vi "Test Set Balance.vi"(8 "error in (no error)":errorcluster, 11 "Test Case In":refnum<class "Account Database Test.lvclass">) -> (0 "error out":errorcluster, 3 "Test Case Out":refnum<class "Account Database Test.lvclass">)   [LabVIEW 2020, in "Account Database Test.lvclass"]
uses:
  Account Database Test.lvclass
  C:/Program Files (x86)/National Instruments/LabVIEW 2020/vi.lib/Astemes/LUnit/Test Case.lvclass
  <vilib>/Astemes/LUnit/Test Case.lvclass/Test Case.ctl
  323c7dbb-e18d-4710-9182-97262e8b68d0.vi
  <vilib>/Astemes/LUnit/Palette/Pass.vi
  <vilib>/Astemes/LUnit/Palette/Fail.vi
  <vilib>/Astemes/LUnit/Compare Variants.vi
  <vilib>/Astemes/LUnit/Describe Comparison.vi
  <vilib>/Astemes/LUnit/Set Assertion Type.vi
  <vilib>/Astemes/LUnit/Add test result.vi
  <vilib>/Astemes/LUnit/Variant to string.vi
  <vilib>/Astemes/LUnit/LUnit Record Assertion Result.vi
  <vilib>/Astemes/LUnit/LUnit Aggregate Assertion Results.vi
  <vilib>/Astemes/LUnit/Method Result/LUnit Merge Status.vi
  <vilib>/Astemes/LUnit/LUnit Concatenate result strings.vi
  <vilib>/Utility/Data Type/Get Type Information.vi
  <vilib>/Utility/LVClass/Get LV Class Name.vi
  Account Database/Account Database.lvclass
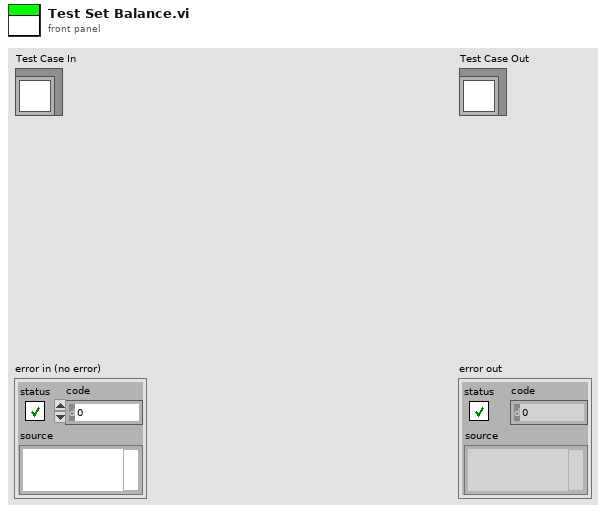
[diagram p1: front panel]
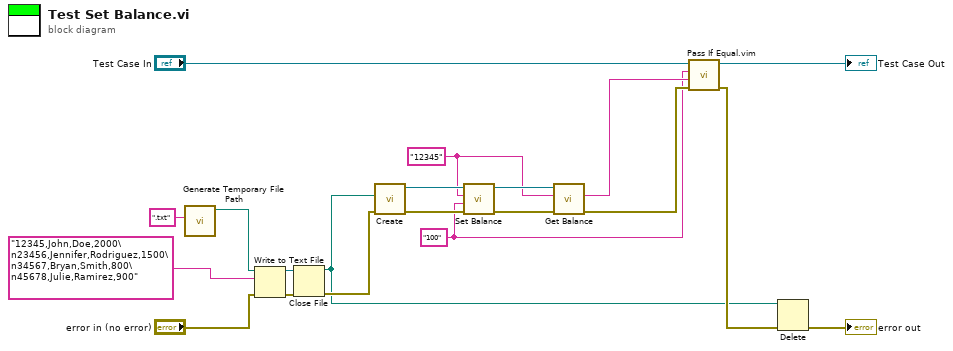
[diagram p0: block diagram]
diagram:
  w4 = "100" ("Account Balance")
  w5 = "12345" ("Account Number")
  n1 = call <vilib>:"Generate Temporary File Path.vi"("Temporary File Extension (tmp)"=".txt") -> ("Unique Temporary File Path"=w12:path)  [unwired: 9 in, 1 out]
  n2 = Write to Text File(file (use dialog)=w12, text="12345,John,Doe,2000\n23456,Jennifer,Rodriguez,1500\n34567,Bryan,Smith,800\n45678,Julie,Ramirez,900", error in="error in (no error)") -> (refnum out=w10:refnum<file>, error out=w11:errorcluster)  [unwired: 1 in, 1 out]
  n3 = Close File(refnum=w10, error in=w11) -> (path=w1:path, error out=w3:errorcluster)
  n4 = call "Create.vi"("error in (no error)"=w3, "Data File"=w1) -> ("error out"=w17:errorcluster, "Account Database out"=w7:refnum<class "Account Database.lvclass">)  [unwired: 8 in]
  n5 = call "Set Balance.vi"("error in (no error)"=w17, "Account Balance"=w4, "Account Number"=w5, "Account Database in"=w7) -> ("error out"=w8:errorcluster, "Account Database out"=w6:refnum<class "Account Database.lvclass">)  [unwired: 6 in]
  n6 = call "Get Balance.vi"("error in (no error)"=w8, "Account Number"=w5, "Account Database in"=w6) -> ("error out"=w16:errorcluster, "Account Balance"=w15:string)  [unwired: 6 in, 1 out]
  n7 = call "Pass If Equal.vim"("error in (no error)"=w16, "Actual"=w15, "Expected"=w4, "LUnit Test Case In"="Test Case In") -> ("error out"=w19:errorcluster, "LUnit Test Case Out"=→"Test Case Out":refnum<class "Account Database Test.lvclass">)  [unwired: 6 in]
  n8 = Delete(path (use dialog)=w1, error in=w19) -> (error out=→"error out":errorcluster)  [unwired: 3 in, 2 out]
